vi "Prepare_Sinus_Waveform_subVI.vi"(8 "error in":errorcluster, 9 "Amplitude":dbl=1.0, 10 "DAQ AO Sinus Config":T1={"Samples"=-10, "Cycles"=-10, "Frequency(Hz)"=-10.0}, 11 "AO Physical Channel":tag) -> (0 "error out":errorcluster, 2 "Waveform":waveform(dbl), 3 "task out":refnum<k21>)   [LabVIEW 2020]
doc: "This Vi prepares waveform for Analog Output DAQ signal generator."
uses:
  Type Definitions/DAQ AO Sinus Config.ctl
  <vilib>/DAQmx/write.llb/DAQmx Write (Analog Wfm 1Chan NSamp).vi
  <vilib>/DAQmx/create/channels.llb/DAQmx Create Channel (AO-Voltage-Basic).vi
  <vilib>/DAQmx/configure/timing.llb/DAQmx Timing (Use Waveform).vi
  <vilib>/DAQmx/miscellaneous.llb/DAQmx Fill In Error Info.vi
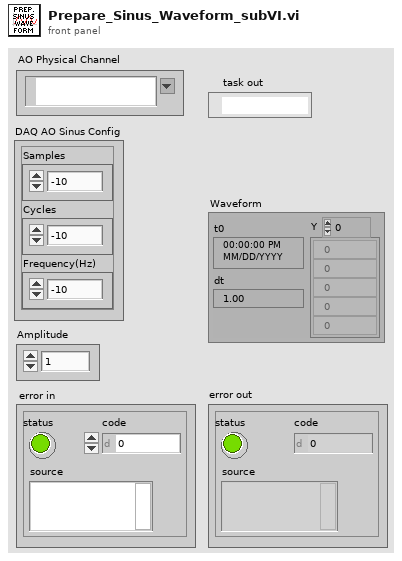
[diagram p1: front panel]
types:
  T1 = typedef "DAQ AO Sinus Config.ctl" = cluster{"Samples":i32, "Cycles":i32, "Frequency(Hz)":dbl}
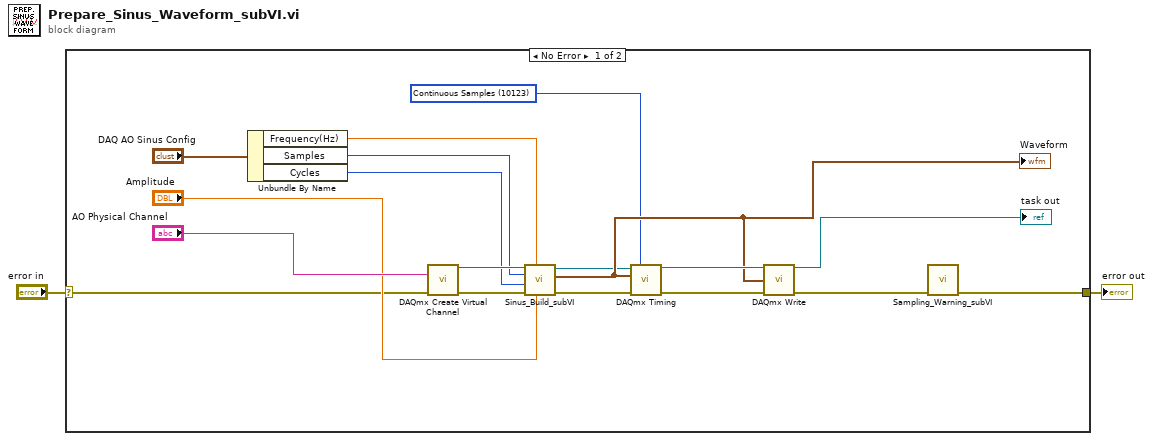
[diagram p0: block diagram]
diagram:
  n1 = case shown="No Error" "error in" {
    selector: "error in" -> [w3 w21]
    tunnel: [w19 w21] -> w2
    frame No Error {
      w5 = 10123 items=["Finite Samples"=10178, "Continuous Samples"=10123, "Hardware Timed Single Point"=12522] ("sample mode")
      n2 = Unbundle By Name("DAQ AO Sinus Config") -> ("Frequency(Hz)"=w11:dbl, "Samples"=w10:i32, "Cycles"=w9:i32)
      n3 = call-poly <vilib>:"DAQmx Create Virtual Channel.vi"("physical channels"="AO Physical Channel", "error in"=w3) -> ("task out"=w17:refnum<k21>, "error out"=w15:errorcluster)  [unwired: 12 in]
      n4 = call "Sinus_Build_subVI.vi"("Amplitude"="Amplitude", "Desired Frequency"=w11, "error in"=w15, "Cycles per Buffer"=w9, "Samples per Buffer"=w10, "task in"=w17) -> ("error out"=w16:errorcluster, "Waveform"=w7:waveform(dbl), "task out"=w6:refnum<k21>)  [unwired: 3 in]
      "Waveform" <- w7
      n5 = call-poly <vilib>:"DAQmx Timing.vi"("task/channels in"=w6, "sample mode"=w5, "waveform"=w7, "error in"=w16) -> ("task out"=w14:refnum<k21>, "error out"=w18:errorcluster)  [unwired: 10 in]
      n6 = call-poly <vilib>:"DAQmx Write.vi"("task/channels in"=w14, "data"=w7, "error in"=w18) -> ("task out"=→"task out":refnum<k21>, "error out"=w20:errorcluster)  [unwired: 10 in, 1 out]
      n7 = call "Sampling_Warning_subVI.vi"("error in (no error)"=w20) -> ("error out"=w19:errorcluster)  [unwired: 10 in]
    }
    frame Error {
    }
  }
  "error out" <- w2
